vi "RPM.vi"(11 "Input":i32) -> (3 "RPM":dbl)   [LabVIEW 2023, in "Test_Libraries.lvlib"]
uses:
  Proyecto/Test_Libraries.lvlib
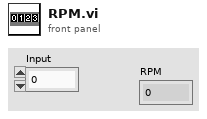
[diagram p1: front panel]
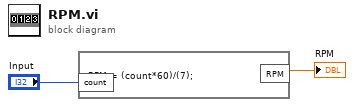
[diagram p0: block diagram]
diagram:
  n1 = formula code="RPM = (count*60)/(7);"("count"="Input") -> ("RPM"=→"RPM":dbl)
